vi "labview-data.vi"() -> ()   [LabVIEW 2023]
panel:
  in  "error in (no error) 2":errorcluster
  out "error out 2":errorcluster
  in  "Tab Control":enum32{"HOME", "AUTO-MODE", "MACHINE-OPERATION"}(tab)
  in  "Spray-Pump":i32
  out "?":i32
  in  "Scrubber-Pump":i32
  in  "Inlet-Temperature":i32
  in  "Bed-Temperature":i32
  in  "Exhaust-Temperature":i32
  out "?":i32
  out "?":i32
  out "?":i32
  out "?":i32
  in  "Spray Gun-1 Pressure":i32
  in  "Spray Gun-2 Pressure":i32
  in  "Spray Gun-3 Pressure":i32
  out "?":i32
  out "?":i32
  out "?":i32
  in  "ON/OFF":bool
  in  "module path":path
  in  "module path 2":path
  out "?":i32
  out "?":i32
  in  "MACHINE PAUSE":i32
  in  "MACHINE OFF TIME":i32
  out "?":i32
  in  "MACHINE ON TIME":i32
  in  "ON/OFF 2":bool caption="ON/OFF"
  out "error out":errorcluster
  in  "error in (no error)":errorcluster
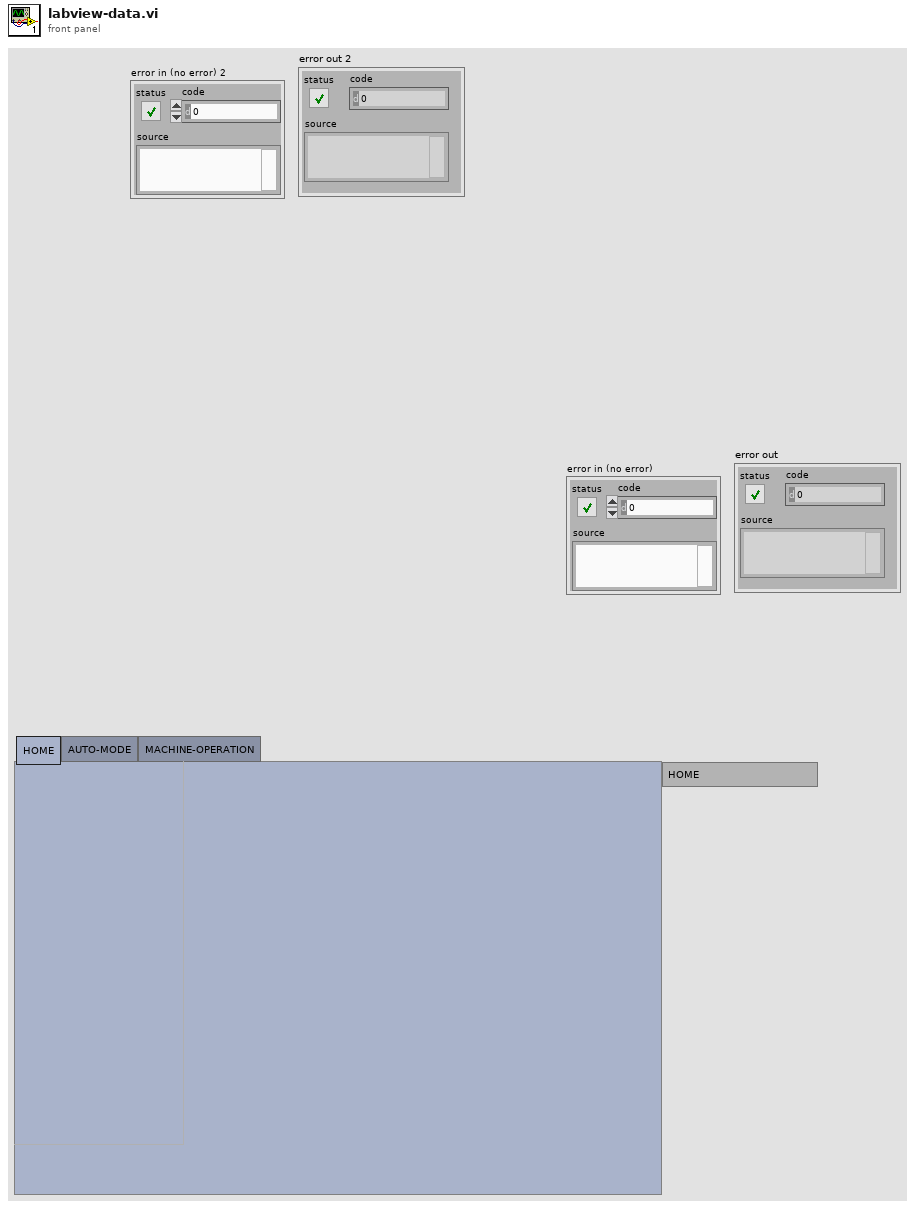
[diagram p1: front panel]
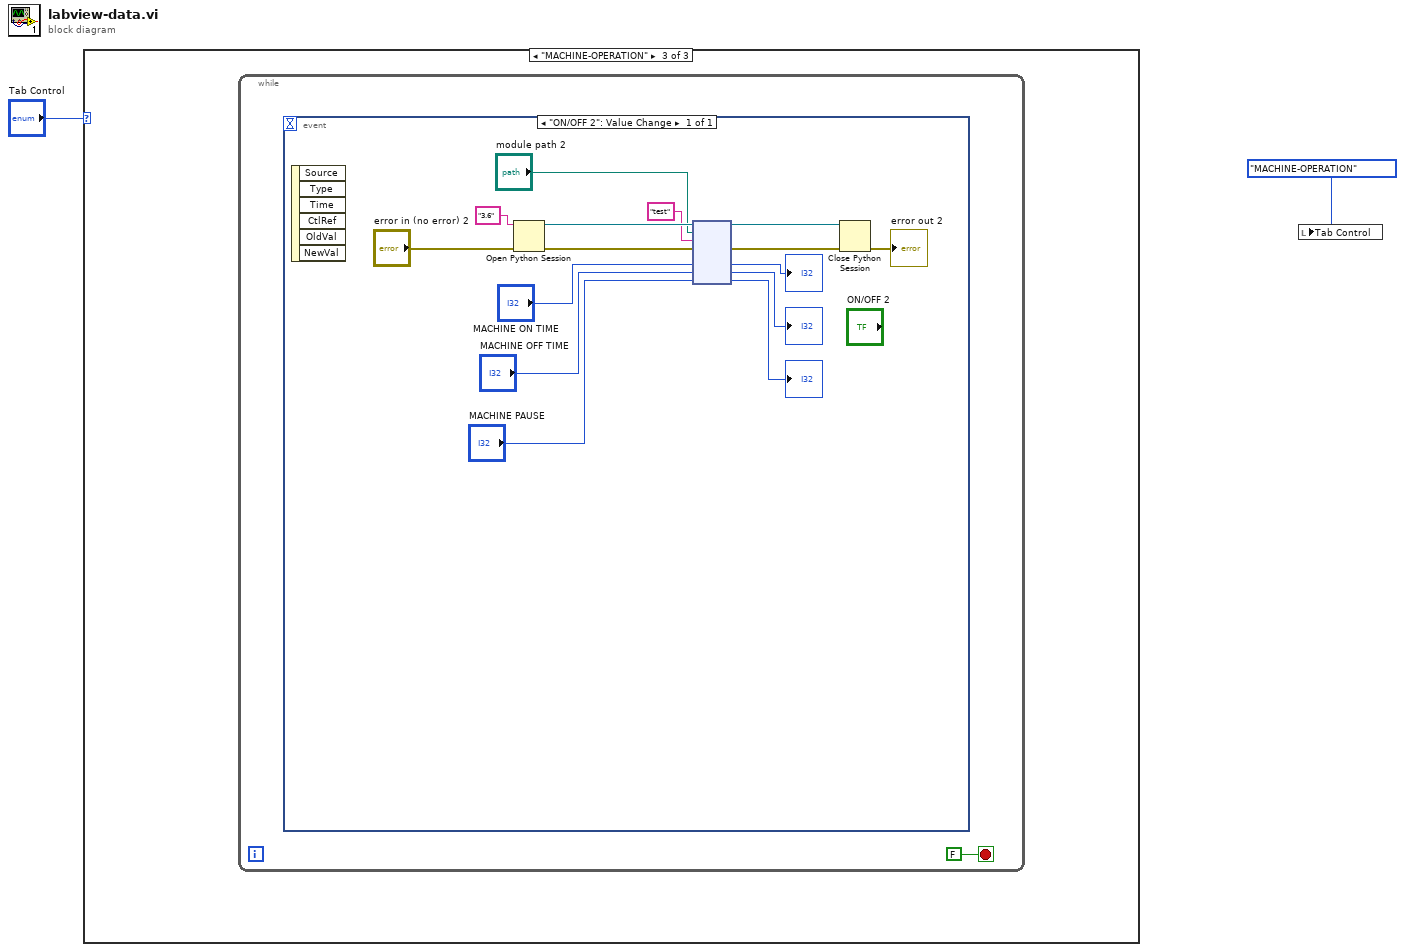
[diagram p0: block diagram]
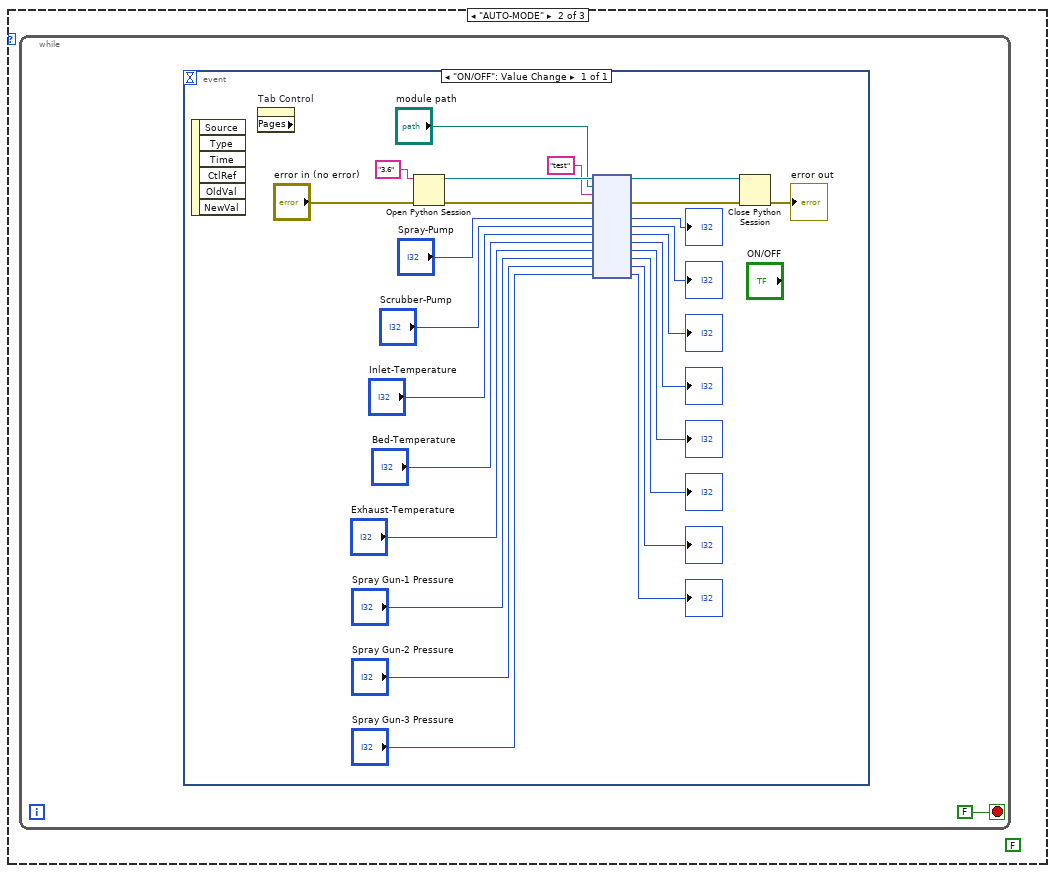
[diagram p3: hidden frame]
diagram:
  n1 = case shown="\"MACHINE-OPERATION\"" "Tab Control" {
    frame "HOME", Default {
    }
    frame "AUTO-MODE" {
      (unwired) FALSE
      n2 = while {
        stop <- FALSE stop-if-true
        n3 = event shown="[0] \"ON/OFF\": Value Change" {
          selector: _ -> [_]
          dyn-events: _ -> [_]
          timeout: _ -> [_]
          event "ON/OFF": Value Change {
            n4 = event-data() -> ()  [unwired: 1 in, 6 out]
            n5 = property on="Tab Control" class="TabCtl (strict)" props=["Pages"]() -> ()  [unwired: 2 in, 3 out]
            n6 = Open Python Session(python version="3.6" ("Python version"), 3:"error in (no error)") -> (session out=w26:refnum<k35>, error out=w25:errorcluster)  [unwired: 1 in]
            n7 = node(w26, "module path", "test" ("function name"), w25, "Spray-Pump", "Scrubber-Pump", "Inlet-Temperature", "Bed-Temperature", "Exhaust-Temperature", "Spray Gun-1 Pressure", "Spray Gun-2 Pressure", "Spray Gun-3 Pressure") -> (w23:refnum<k35>, w22:errorcluster, →"?":i32, →"?":i32, →"?":i32, →"?":i32, →"?":i32, →"?":i32, →"?":i32, →"?":i32)  [unwired: 2 in, 2 out]
            n8 = Close Python Session(session in=w23, error in=w22) -> (11:→"error out":errorcluster)
          }
        }
      }
    }
    frame "MACHINE-OPERATION" {
      n9 = while {
        stop <- FALSE stop-if-true
        n10 = event shown="[0] \"ON/OFF 2\": Value Change" {
          selector: _ -> [_]
          dyn-events: _ -> [_]
          timeout: _ -> [_]
          event "ON/OFF 2": Value Change {
            n11 = event-data() -> ()  [unwired: 1 in, 6 out]
            n12 = Open Python Session(python version="3.6" ("Python version"), 3:"error in (no error) 2") -> (session out=w42:refnum<k35>, error out=w41:errorcluster)  [unwired: 1 in]
            n13 = node(w42, "module path 2", "test" ("function name"), w41, "MACHINE ON TIME", "MACHINE OFF TIME", "MACHINE PAUSE") -> (w39:refnum<k35>, w38:errorcluster, →"?":i32, →"?":i32, →"?":i32)  [unwired: 2 in, 2 out]
            n14 = Close Python Session(session in=w39, error in=w38) -> (11:→"error out 2":errorcluster)
          }
        }
      }
    }
  }
  n15 = local write "Tab Control"(enum32{"HOME", "AUTO-MODE", "MACHINE-OPERATION"}."MACHINE-OPERATION" ("Tab Control")) -> ()
